vi "DSF.Engine.Plugin.Rx.vi"(8 "error in (no error)":errorcluster, 10 "Transfer Group in":refnum<class "DSF.Engine.Transfer Group.lvclass">, 11 "GE Reflective Memory Plugin in":refnum<class "DSF.Plugin.GE Reflective Memory.lvclass">) -> (0 "error out":errorcluster, 2 "Transfer Group out":refnum<class "DSF.Engine.Transfer Group.lvclass">, 3 "GE Reflective Memory Plugin out":refnum<class "DSF.Plugin.GE Reflective Memory.lvclass">)   [LabVIEW 2017, in "DSF.Plugin.GE Reflective Memory.lvclass"]
uses:
  DSF.Plugin.GE Reflective Memory.lvclass
  Engine/Classes/Transfer/DSF.Engine.Transfer Group.lvclass
  Engine/Classes/Plugin/Plugin.lvclass
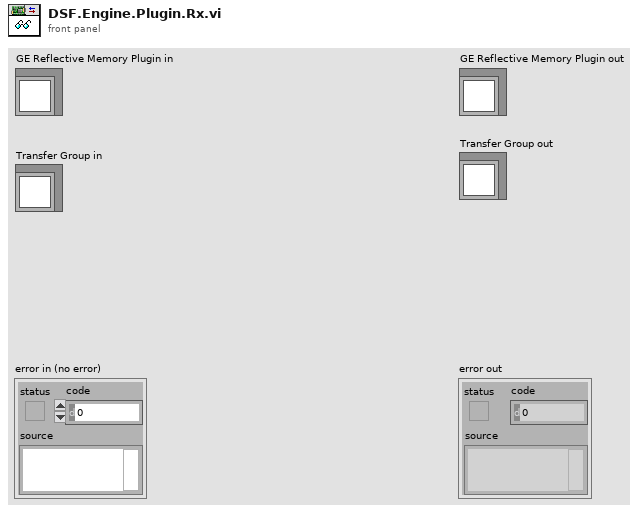
[diagram p1: front panel]
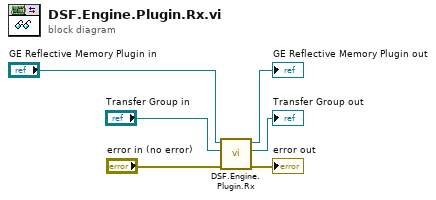
[diagram p0: block diagram]
diagram:
  n1 = call-parent "DSF.Engine.Plugin.Rx.vi"("error in (no error)"="error in (no error)", "Transfer Group in"="Transfer Group in", "Plugin in"="GE Reflective Memory Plugin in") -> ("error out"=→"error out":errorcluster, "Transfer Group out"=→"Transfer Group out":refnum<class "DSF.Engine.Transfer Group.lvclass">, "Plugin out"=→"GE Reflective Memory Plugin out":refnum<class "DSF.Plugin.GE Reflective Memory.lvclass">)  [unwired: 6 in]
